vi "3D-Limit Collect.vi"(11 "Limit Input":string[][](table)) -> (3 "Limit Output":string[](array[string]))   [LabVIEW 2015]
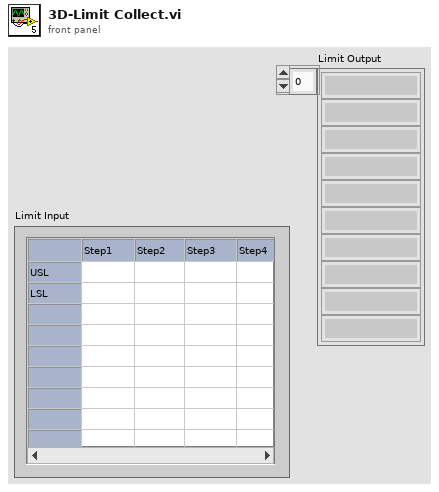
[diagram p1: front panel]
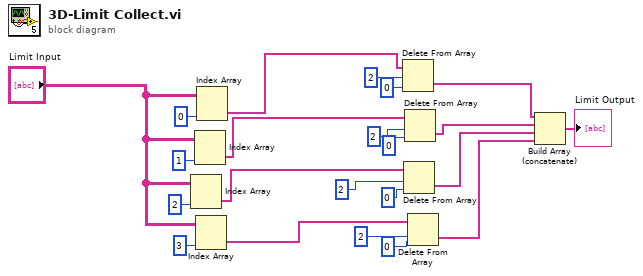
[diagram p0: block diagram]
diagram:
  n1 = Index Array(array="Limit Input", index (col)=2 ("禁用的索引 (列)")) -> (element=w7:string[])  [unwired: 1 in]
  n2 = Index Array(array="Limit Input", index (col)=1 ("禁用的索引 (列)")) -> (element=w8:string[])  [unwired: 1 in]
  n3 = Index Array(array="Limit Input", index (col)=3 ("禁用的索引 (列)")) -> (element=w6:string[])  [unwired: 1 in]
  n4 = Index Array(array="Limit Input", index (col)=0 ("禁用的索引 (列)")) -> (element=w10:string[])  [unwired: 1 in]
  n5 = Delete From Array(array=w10, length=2 ("长度"), index=0 ("索引")) -> (deleted portion=w2:string[])  [unwired: 1 out]
  n6 = Delete From Array(array=w7, length=2 ("长度"), index=0 ("禁用的索引 (列)")) -> (deleted portion=w17:string[])  [unwired: 1 out]
  n7 = Delete From Array(array=w8, length=2 ("长度"), index=0 ("禁用的索引 (列)")) -> (deleted portion=w18:string[])  [unwired: 1 out]
  n8 = Delete From Array(array=w6, length=2 ("长度"), index=0 ("禁用的索引 (列)")) -> (deleted portion=w16:string[])  [unwired: 1 out]
  n9 = Build Array (concatenate)(w2, w18, w17, w16) -> (→"Limit Output":string[])
